vi "DAQ 실습_종합.vi"() -> ()   [LabVIEW 2020]
uses:
  <vilib>/DAQmx/create/channels.llb/DAQmx Create Channel (AI-Voltage-Basic).vi
  <vilib>/DAQmx/read.llb/DAQmx Read (Analog 1D DBL 1Chan NSamp).vi
  <vilib>/DAQmx/configure/timing.llb/DAQmx Timing (Sample Clock).vi
  <vilib>/DAQmx/read.llb/DAQmx Read (Analog DBL 1Chan 1Samp).vi
  <vilib>/DAQmx/create/channels.llb/DAQmx Create Channel (AO-Voltage-Basic).vi
  <vilib>/DAQmx/configure/timing.llb/DAQmx Timing (Use Waveform).vi
  <vilib>/DAQmx/write.llb/DAQmx Write (Analog Wfm 1Chan NSamp).vi
  <vilib>/DAQmx/write.llb/DAQmx Write (Analog Wfm 1Chan 1Samp).vi
panel:
  in  "정지 2":bool
  out "x-y 3":u32
  out "x-y 2":u32
  out "x*y":dbl[](graph)
  out "크기":i32
  out "x-y":u32
  in  "정지":bool
  out "data":dbl caption="데이터" format="%0.2f"
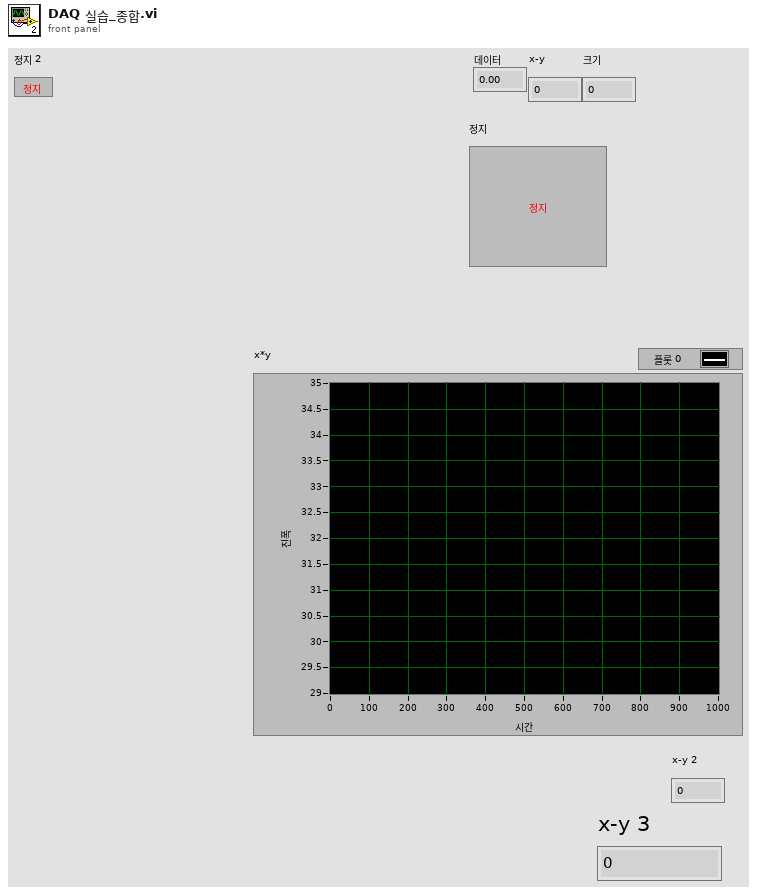
[diagram p1: front panel]
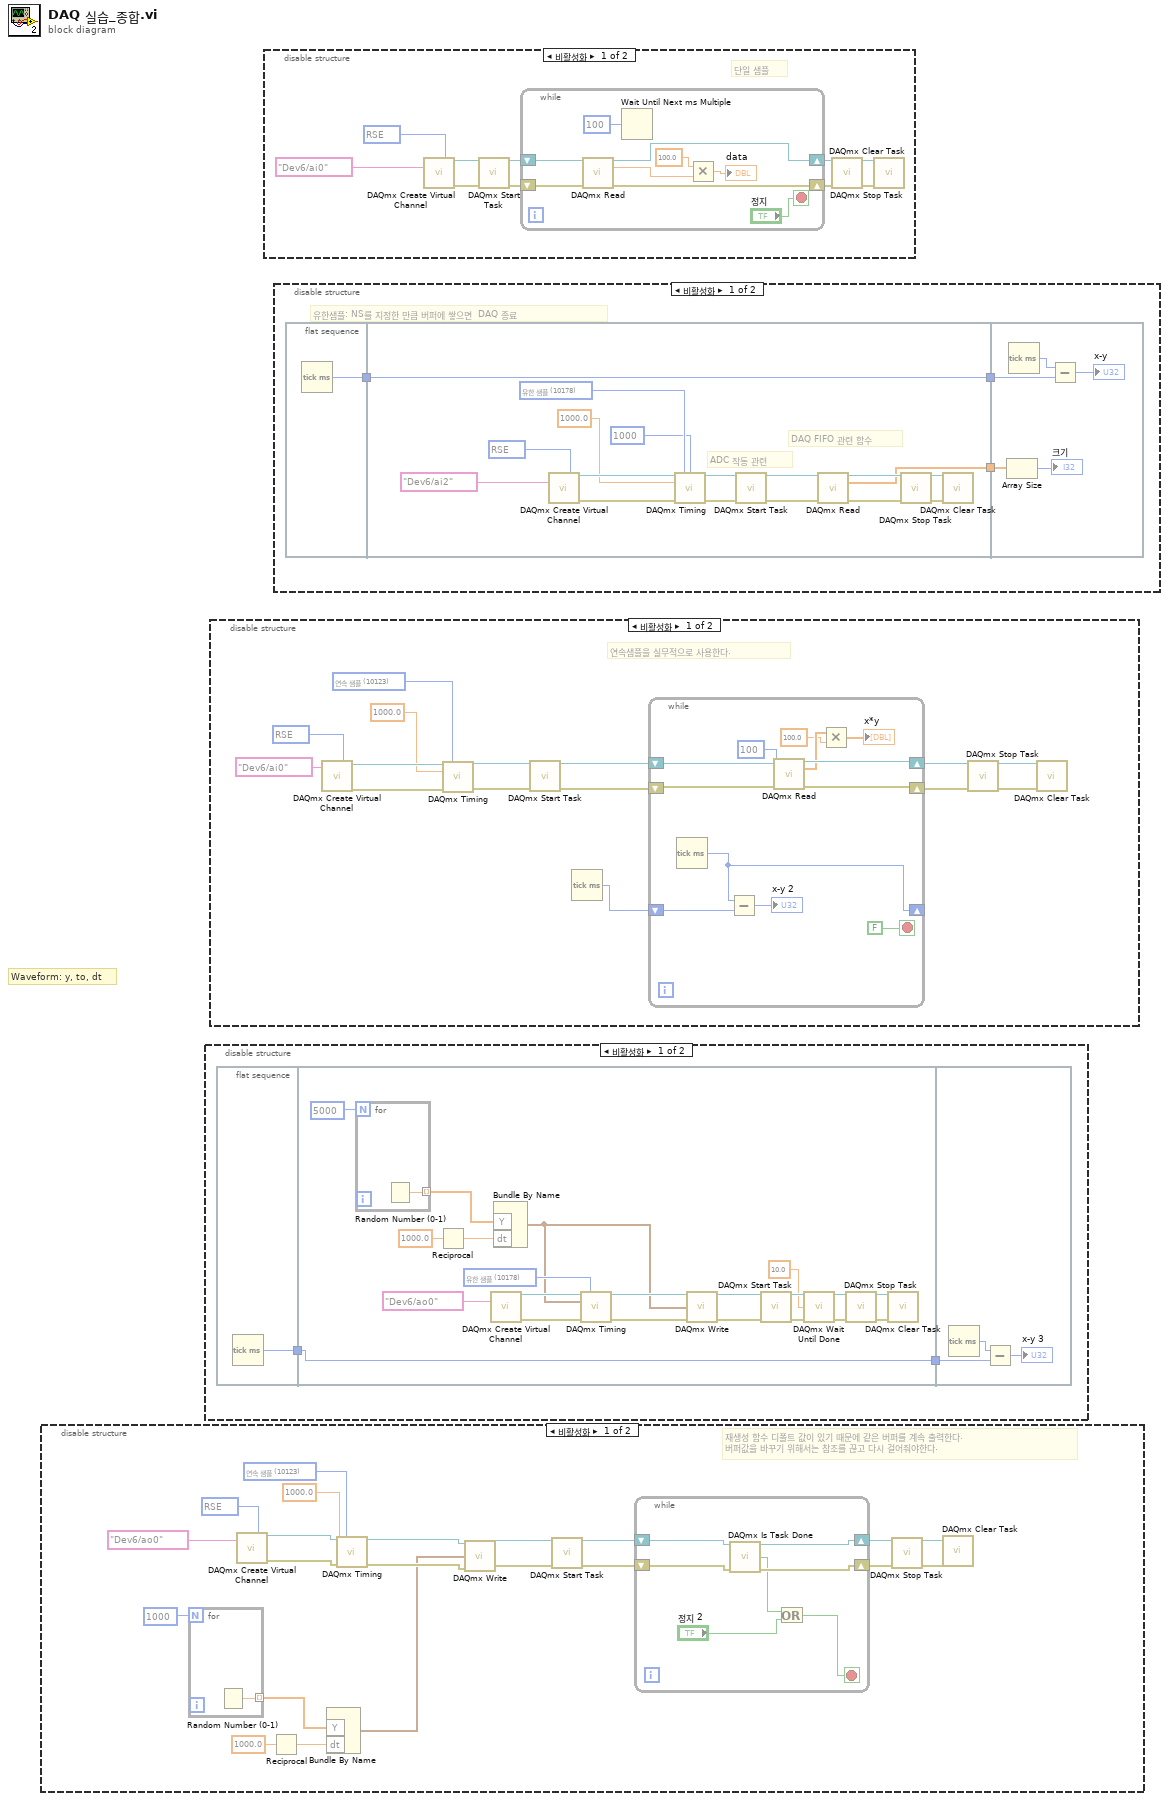
[diagram p0: block diagram]
diagram:
  # "Waveform: y, to, dt"
  n1 = disable-structure shown="비활성화" {
    frame Disabled {
      w17 = 10123 items=["유한 샘플"=10178, "연속 샘플"=10123, "하드웨어 타이밍에 의한 단일 포인트"=12522] ("sample mode")
      w20 = 10083 items=["기본"=-1, "RSE"=10083, "차동"=10106, "유사 차동"=12529] ("output terminal configuration")
      # "재생성 함수 디폴트 값이 있기 때문에 같은 버퍼를 계속 출력한다.\n버퍼값을 바꾸기 위해서는 참조를 끊고 다시 걸어줘야한다."
      n2 = for {
        N: 1000 -> [_]
        tunnel: [w29] -> w15 mode=indexing
        n3 = Random Number (0-1)() -> (number: 0 to 1=w29:dbl)
      }
      n4 = call-poly <vilib>:"DAQmx Create Virtual Channel.vi"("output terminal configuration"=w20, "physical channels"=tag "Dev6/ao0") -> ("task out"=w19:refnum<k21>, "error out"=w18:errorcluster)  [unwired: 12 in]
      n5 = Reciprocal(x=1000.0 ("rate")) -> (1/x=w14:dbl)
      n6 = Bundle By Name("Y"=w15, "dt"=w14) -> (w9:waveform(dbl))  [unwired: 1 in]
      n7 = call-poly <vilib>:"DAQmx Timing.vi"("task/channels in"=w19, "sample mode"=w17, "rate"=1000.0, "error in"=w18) -> ("task out"=w11:refnum<k21>, "error out"=w10:errorcluster)  [unwired: 10 in]
      n8 = call-poly <vilib>:"DAQmx Write.vi"("task/channels in"=w11, "data"=w9, "error in"=w10) -> ("task out"=w8:refnum<k21>, "error out"=w7:errorcluster)  [unwired: 10 in, 1 out]
      n9 = call <vilib>:"DAQmx Start Task.vi"("task/channels in"=w8, "error in"=w7) -> ("task out"=w6:refnum<k21>, "error out"=w5:errorcluster)  [unwired: 12 in]
      n10 = while {
        shift-right: [w26] -> w4
        shift-left: w6 -> [w28]
        shift-right: [w25] -> w3
        shift-left: w5 -> [w27]
        stop <- w23 stop-if-true
        n11 = call <vilib>:"DAQmx Is Task Done.vi"("task/channels in"=w28, "error in"=w27) -> ("task out"=w26:refnum<k21>, "task done?"=w22:bool, "error out"=w25:errorcluster)  [unwired: 11 in]
        n12 = Or(x=w22, y="정지 2") -> (x .or. y?=w23:bool)
      }
      n13 = call <vilib>:"DAQmx Stop Task.vi"("task/channels in"=w4, "error in"=w3) -> ("task out"=w2:refnum<k21>, "error out"=w1:errorcluster)  [unwired: 12 in]
      n14 = call <vilib>:"DAQmx Clear Task.vi"("task in"=w2, "error in"=w1) -> ()  [unwired: 13 in, 1 out]
    }
    frame Enabled {
    }
  }
  n15 = disable-structure shown="비활성화" {
    frame Disabled {
      n16 = flat-sequence {
        tunnel: [w32] -> w31
        tunnel: w31 -> [w37]
        tunnel: [w37] -> w30
        tunnel: w30 -> [w56]
        frame #0 {
          n17 = Tick Count (ms)() -> (millisecond timer value=w32:u32)
        }
        frame #1 {
          w49 = 10178 items=["유한 샘플"=10178, "연속 샘플"=10123, "하드웨어 타이밍에 의한 단일 포인트"=12522] ("sample mode")
          n18 = for {
            N: 5000 -> [_]
            tunnel: [w54] -> w34 mode=indexing
            n19 = Random Number (0-1)() -> (number: 0 to 1=w54:dbl)
          }
          n20 = Reciprocal(x=1000.0 ("rate")) -> (1/x=w35:dbl)
          n21 = call-poly <vilib>:"DAQmx Create Virtual Channel.vi"("physical channels"=tag "Dev6/ao0") -> ("task out"=w52:refnum<k21>, "error out"=w51:errorcluster)  [unwired: 13 in]
          n22 = Bundle By Name("Y"=w34, "dt"=w35) -> (w33:waveform(dbl))  [unwired: 1 in]
          n23 = call-poly <vilib>:"DAQmx Timing.vi"("task/channels in"=w52, "sample mode"=w49, "waveform"=w33, "error in"=w51) -> ("task out"=w50:refnum<k21>, "error out"=w48:errorcluster)  [unwired: 10 in]
          n24 = call-poly <vilib>:"DAQmx Write.vi"("task/channels in"=w50, "data"=w33, "error in"=w48) -> ("task out"=w46:refnum<k21>, "error out"=w45:errorcluster)  [unwired: 10 in, 1 out]
          n25 = call <vilib>:"DAQmx Start Task.vi"("task/channels in"=w46, "error in"=w45) -> ("task out"=w44:refnum<k21>, "error out"=w43:errorcluster)  [unwired: 12 in]
          n26 = call <vilib>:"DAQmx Wait Until Done.vi"("task/channels in"=w44, "timeout (sec)"=10.0, "error in"=w43) -> ("task out"=w42:refnum<k21>, "error out"=w41:errorcluster)  [unwired: 11 in]
          n27 = call <vilib>:"DAQmx Stop Task.vi"("task/channels in"=w42, "error in"=w41) -> ("task out"=w40:refnum<k21>, "error out"=w39:errorcluster)  [unwired: 12 in]
          n28 = call <vilib>:"DAQmx Clear Task.vi"("task in"=w40, "error in"=w39) -> ()  [unwired: 13 in, 1 out]
        }
        frame #2 {
          n29 = Tick Count (ms)() -> (millisecond timer value=w57:u32)
          n30 = Subtract(x=w57, y=w56) -> (x-y=→"x-y 3":u32)
        }
      }
    }
    frame Enabled {
    }
  }
  n31 = disable-structure shown="비활성화" {
    frame Disabled {
      w67 = 10123 items=["유한 샘플"=10178, "연속 샘플"=10123, "하드웨어 타이밍에 의한 단일 포인트"=12522] ("sample mode")
      w71 = 10083 items=["기본"=-1, "RSE"=10083, "NRSE"=10078, "차동"=10106, "유사 차동"=12529] ("input terminal configuration")
      # "연속샘플을 실무적으로 사용한다."
      n32 = call-poly <vilib>:"DAQmx Create Virtual Channel.vi"("input terminal configuration"=w71, "physical channels"=tag "Dev6/ai0") -> ("task out"=w70:refnum<k21>, "error out"=w69:errorcluster)  [unwired: 12 in]
      n33 = call-poly <vilib>:"DAQmx Timing.vi"("task/channels in"=w70, "sample mode"=w67, "rate"=1000.0, "error in"=w69) -> ("task out"=w66:refnum<k21>, "error out"=w65:errorcluster)  [unwired: 10 in]
      n34 = call <vilib>:"DAQmx Start Task.vi"("task/channels in"=w66, "error in"=w65) -> ("task out"=w64:refnum<k21>, "error out"=w63:errorcluster)  [unwired: 12 in]
      n35 = Tick Count (ms)() -> (millisecond timer value=w58:u32)
      n36 = while {
        shift-right: [w81] -> w62
        shift-left: w64 -> [w84]
        shift-right: [w82] -> w61
        shift-left: w63 -> [w83]
        shift-right: [w74] -> _
        shift-left: w58 -> [w75]
        stop <- FALSE stop-if-true
        n37 = Tick Count (ms)() -> (millisecond timer value=w74:u32)
        n38 = Subtract(x=w74, y=w75) -> (x-y=→"x-y 2":u32)
        n39 = call-poly <vilib>:"DAQmx Read.vi"("task/channels in"=w84, "number of samples per channel"=100, "error in"=w83) -> ("task out"=w81:refnum<k21>, "data"=w78:dbl[], "error out"=w82:errorcluster)  [unwired: 10 in]
        n40 = Multiply(x=w78, y=100.0) -> (x*y=→"x*y":dbl[])
      }
      n41 = call <vilib>:"DAQmx Stop Task.vi"("task/channels in"=w62, "error in"=w61) -> ("task out"=w60:refnum<k21>, "error out"=w59:errorcluster)  [unwired: 12 in]
      n42 = call <vilib>:"DAQmx Clear Task.vi"("task in"=w60, "error in"=w59) -> ()  [unwired: 13 in, 1 out]
    }
    frame Enabled {
    }
  }
  n43 = disable-structure shown="비활성화" {
    frame Disabled {
      w93 = 10083 items=["기본"=-1, "RSE"=10083, "NRSE"=10078, "차동"=10106, "유사 차동"=12529] ("input terminal configuration")
      # "단일 샘플"
      n44 = call-poly <vilib>:"DAQmx Create Virtual Channel.vi"("input terminal configuration"=w93, "physical channels"=tag "Dev6/ai0") -> ("task out"=w92:refnum<k21>, "error out"=w91:errorcluster)  [unwired: 12 in]
      n45 = call <vilib>:"DAQmx Start Task.vi"("task/channels in"=w92, "error in"=w91) -> ("task out"=w90:refnum<k21>, "error out"=w89:errorcluster)  [unwired: 12 in]
      n46 = while {
        shift-right: [w101] -> w88
        shift-left: w90 -> [w103]
        shift-right: [w100] -> w87
        shift-left: w89 -> [w102]
        stop <- "정지" stop-if-true
        n47 = call-poly <vilib>:"DAQmx Read.vi"("task/channels in"=w103, "error in"=w102) -> ("task out"=w101:refnum<k21>, "data"=w99:dbl, "error out"=w100:errorcluster)  [unwired: 11 in]
        n48 = Wait Until Next ms Multiple(millisecond multiple=u32 100 ("ms 배수")) -> ()  [unwired: 1 out]
        n49 = Multiply(x=100.0, y=w99) -> (x*y=→"data":dbl)
      }
      n50 = call <vilib>:"DAQmx Stop Task.vi"("task/channels in"=w88, "error in"=w87) -> ("task out"=w86:refnum<k21>, "error out"=w85:errorcluster)  [unwired: 12 in]
      n51 = call <vilib>:"DAQmx Clear Task.vi"("task in"=w86, "error in"=w85) -> ()  [unwired: 13 in, 1 out]
    }
    frame Enabled {
    }
  }
  n52 = disable-structure shown="비활성화" {
    frame Disabled {
      # "유한샘플: NS를 지정한 만큼 버퍼에 쌓으면  DAQ 종료"
      n53 = flat-sequence {
        tunnel: [w107] -> w106
        tunnel: w106 -> [w109]
        tunnel: [w109] -> w105
        tunnel: [w108] -> w104
        tunnel: w105 -> [w128]
        tunnel: w104 -> [w126]
        frame #0 {
          n54 = Tick Count (ms)() -> (millisecond timer value=w107:u32)
        }
        frame #1 {
          w119 = 10178 items=["유한 샘플"=10178, "연속 샘플"=10123, "하드웨어 타이밍에 의한 단일 포인트"=12522] ("sample mode")
          w123 = 10083 items=["기본"=-1, "RSE"=10083, "NRSE"=10078, "차동"=10106, "유사 차동"=12529] ("input terminal configuration")
          # "ADC 작동 관련"
          # "DAQ FIFO 관련 함수"
          n55 = call-poly <vilib>:"DAQmx Create Virtual Channel.vi"("input terminal configuration"=w123, "physical channels"=tag "Dev6/ai2") -> ("task out"=w122:refnum<k21>, "error out"=w121:errorcluster)  [unwired: 12 in]
          n56 = call-poly <vilib>:"DAQmx Timing.vi"("task/channels in"=w122, "sample mode"=w119, "samples per channel"=1000, "rate"=1000.0, "error in"=w121) -> ("task out"=w117:refnum<k21>, "error out"=w116:errorcluster)  [unwired: 9 in]
          n57 = call <vilib>:"DAQmx Start Task.vi"("task/channels in"=w117, "error in"=w116) -> ("task out"=w115:refnum<k21>, "error out"=w114:errorcluster)  [unwired: 12 in]
          n58 = call-poly <vilib>:"DAQmx Read.vi"("task/channels in"=w115, "error in"=w114) -> ("task out"=w113:refnum<k21>, "data"=w108:dbl[], "error out"=w112:errorcluster)  [unwired: 11 in]
          n59 = call <vilib>:"DAQmx Stop Task.vi"("task/channels in"=w113, "error in"=w112) -> ("task out"=w111:refnum<k21>, "error out"=w110:errorcluster)  [unwired: 12 in]
          n60 = call <vilib>:"DAQmx Clear Task.vi"("task in"=w111, "error in"=w110) -> ()  [unwired: 13 in, 1 out]
        }
        frame #2 {
          n61 = Array Size(array=w126) -> (size(s)=→"크기":i32)
          n62 = Tick Count (ms)() -> (millisecond timer value=w129:u32)
          n63 = Subtract(x=w129, y=w128) -> (x-y=→"x-y":u32)
        }
      }
    }
    frame Enabled {
    }
  }
